vi "RTB_MODCA.vi"() -> ()   [LabVIEW 2013]
uses:
  <vilib>/Analysis/baseanly.llb/Mean (DBL).vi
  <vilib>/Analysis/NI_AALPro.lvlib
  <vilib>/Analysis/NI_AALBase.lvlib
panel:
  out "mean":dbl
  in  "x":dbl=50.0 format="%#_13g"
  out "Lower":dbl
  out "Upper":dbl
  out "Boolean 3":bool
  out "output":dbl[](array[numeric])
  out "size":i32
  in  "Reset":bool
  out "Graph":dbl[](graph)
  in  "stop":bool
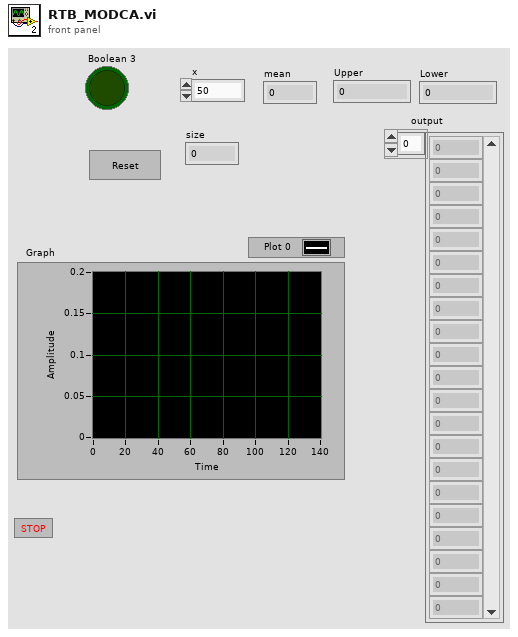
[diagram p1: front panel]
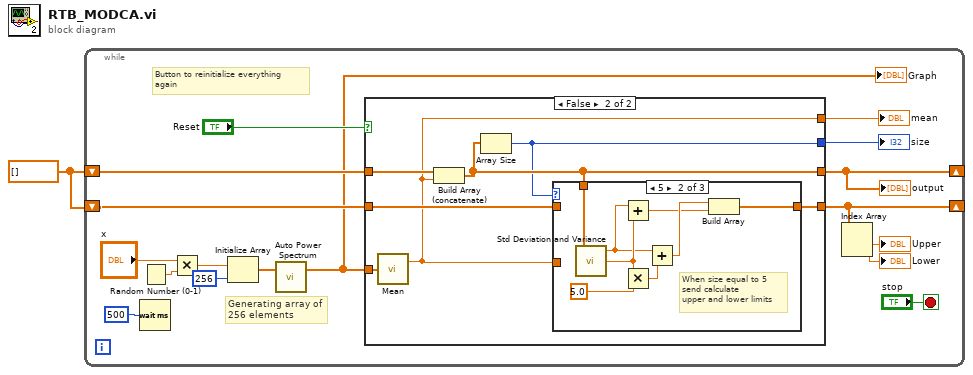
[diagram p0: block diagram]
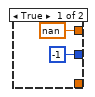
[diagram p2: hidden frame]
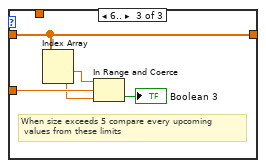
[diagram p4: hidden frame]
diagram:
  w1 = dbl[] []
  n1 = while {
    shift-right: [w5] -> _
    shift-left: w1 -> [w10]
    shift-right: [w8] -> _
    shift-left: w1 -> [w9]
    stop <- "stop" stop-if-true
    # "Generating array of \n256 elements"
    # "Button to reinitialize everything \nagain"
    n2 = Wait (ms)(milliseconds to wait=u32 500) -> ()  [unwired: 1 out]
    n3 = Random Number (0-1)() -> (number: 0 to 1=w13:dbl)
    n4 = Multiply(x="x", y=w13) -> (x*y=w11:dbl)
    n5 = Initialize Array(w11, 256 ("dimension size")) -> (w16:dbl[])
    n6 = call <vilib>:"Auto Power Spectrum.vi"("Signal (V)"=w16) -> ("Power Spectrum (V^2 rms)"=w2:dbl[])  [unwired: 1 in, 1 out]
    "Graph" <- w2
    n7 = case shown="False" "Reset" {
      tunnel: w2 -> [_ w27]
      tunnel: w10 -> [_ w26]
      tunnel: [_ w25] -> w5
      tunnel: w9 -> [_ w23]
      tunnel: [_ w24] -> w8
      tunnel: [-1 w22] -> w4
      tunnel: [nan ("mean") w21] -> w3
      frame True {
      }
      frame False {
        n8 = call-poly <vilib>:"Mean.vi"("X"=w27) -> ("mean"=w21:dbl)  [unwired: 1 out]
        n9 = Build Array (concatenate)(w26, w21) -> (w25:dbl[])
        n10 = Array Size(array=w25) -> (size(s)=w22:i32)
        n11 = case shown="5" w22 {
          tunnel: w25 -> [_ w35 _]
          tunnel: w21 -> [_ _ w40]
          tunnel: [w28 w33 w39] -> w24
          tunnel: w23 -> [w28 _ w39]
          frame Default {
          }
          frame 5 {
            # "When size equal to 5\nsend calculate \nupper and lower limits"
            n12 = call <vilib>:"Std Deviation and Variance.vi"("X"=w35) -> ("mean"=w29:dbl, "standard deviation"=w30:dbl)  [unwired: 1 in, 1 out]
            n13 = Add(x=w29, y=w30) -> (x+y=w31:dbl)
            n14 = Multiply(x=w30, y=5.0) -> (x*y=w36:dbl)
            n15 = Add(x=w29, y=w36) -> (x+y=w32:dbl)
            n16 = Build Array(w32, w31) -> (w33:dbl[])
          }
          frame 6.. {
            # "When size exceeds 5 compare every upcoming\n values from these limits"
            n17 = Index Array(array=w39) -> (element #1=w38:dbl, element #2=w37:dbl)  [unwired: 2 in]
            n18 = In Range and Coerce(upper limit=w38, x=w40, lower limit=w37) -> (In Range?=→"Boolean 3":bool)  [unwired: 1 out]
          }
        }
      }
    }
    "output" <- w5
    "size" <- w4
    "mean" <- w3
    n19 = Index Array(array=w8) -> (element #1=→"Upper":dbl, element #2=→"Lower":dbl)  [unwired: 2 in]
  }
